vi "PhotonPipelineMetadata_Equals.vi"(9 "Other PhotonPipelineMetadata":T1={"CaptureTimestampMicros"=-1, "PublishTimestampMicros"=-1, "SequenceID"=-1, "TimeSinceLastPong"=9999999999}, 11 "PhotonPipelineMetadata":T1={"CaptureTimestampMicros"=-1, "PublishTimestampMicros"=-1, "SequenceID"=-1, "TimeSinceLastPong"=9999999999}) -> (3 "Equal":bool)   [LabVIEW 2019, in "PhotonVisionLib.lvlib"]
doc: "Determines if two PipelineMetadata clusters are equal.\n\nInputs:\n - PipelineMetadata -- PipelineMetadata cluster.\n - Other PipelineMetadata -- Other Pipelinemetadata cluster.\n\nOutputs:\n - Equal -- Returns TRUE, if both pipeline metadata clusters are equal.."
uses:
  PhotonVisionLib.lvlib
  TypeDef/PhotonPipelineMetadataType.ctl
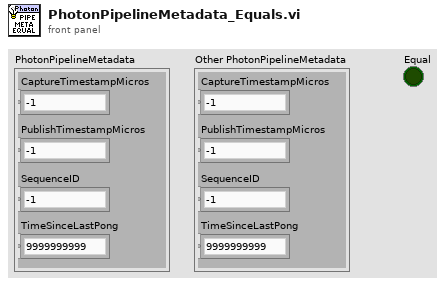
[diagram p1: front panel]
types:
  T1 = typedef "PhotonVisionLib.lvlib/PhotonPipelineMetadataType.ctl" = cluster{"CaptureTimestampMicros":i64, "PublishTimestampMicros":i64, "SequenceID":i64, "TimeSinceLastPong":i64}
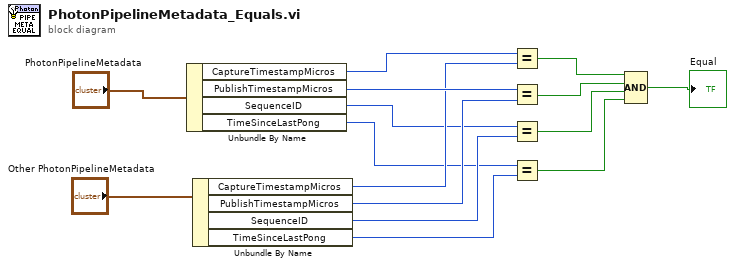
[diagram p0: block diagram]
diagram:
  n1 = Unbundle By Name("PhotonPipelineMetadata") -> ("CaptureTimestampMicros"=w13:i64, "PublishTimestampMicros"=w12:i64, "SequenceID"=w6:i64, "TimeSinceLastPong"=w4:i64)
  n2 = Unbundle By Name("Other PhotonPipelineMetadata") -> ("CaptureTimestampMicros"=w11:i64, "PublishTimestampMicros"=w10:i64, "SequenceID"=w5:i64, "TimeSinceLastPong"=w3:i64)
  n3 = Equal?(x=w13, y=w11) -> (x = y?=w9:bool)
  n4 = Equal?(x=w12, y=w10) -> (x = y?=w8:bool)
  n5 = Equal?(x=w6, y=w5) -> (x = y?=w7:bool)
  n6 = Equal?(x=w4, y=w3) -> (x = y?=w2:bool)
  n7 = Compound Arithmetic op=AND(w9, w8, w7, w2) -> (→"Equal":bool)
